vi "frontsB_ext.vi"(5 "NOT IN OLD":bool[](array[boolean]), 7 "IN":bool[](array[boolean])) -> (1 "NOT IN":bool[](array[boolean]), 2 "FALL":bool[](array[boolean]), 3 "RAISE":bool[](array[boolean]))   [LabVIEW 2019, in "Logik.lvlib"]
uses:
  Logik.lvlib
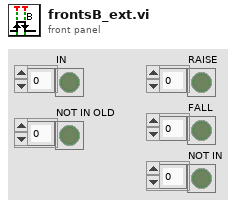
[diagram p1: front panel]
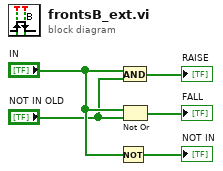
[diagram p0: block diagram]
diagram:
  n1 = Not(x="IN") -> (.not. x?=→"NOT IN":bool[])
  n2 = And(x="IN", y="NOT IN OLD") -> (x .and. y?=→"RAISE":bool[])
  n3 = Not Or(1:"NOT IN OLD", 2:"IN") -> (0:→"FALL":bool[])
